vi "RM.forceAddReservation.vi"(5 "Resource Type":T1, 7 "Direction":T2, 8 "error in":errorcluster, 9 "reserver":string, 10 "name in bitfile":string, 11 "reservation DB in":variant) -> (0 "error out":errorcluster, 1 "replaced":bool, 3 "reservation DB out":variant)   [LabVIEW 2016, in "FPGA Addon Shared.lvlib"]
uses:
  FPGA Addon Shared.lvlib
  RM.resourceDirection.ctl
  RM.resourceType.ctl
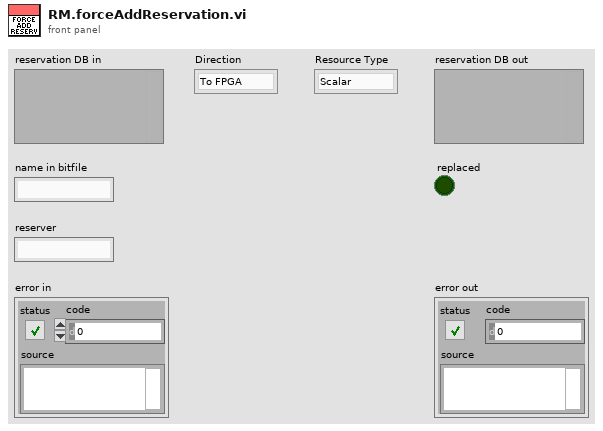
[diagram p1: front panel]
types:
  T1 = typedef "FPGA Addon Shared.lvlib/RM.resourceType.ctl" = enum16{"Scalar", "Waveform"}
  T2 = typedef "FPGA Addon Shared.lvlib/RM.resourceDirection.ctl" = enum16{"To FPGA", "From FPGA"}
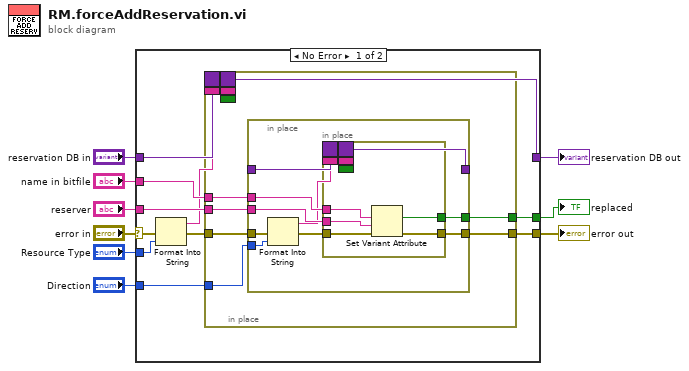
[diagram p0: block diagram]
diagram:
  n1 = case shown="No Error" "error in" {
    selector: "error in" -> [w12 w46]
    tunnel: "reservation DB in" -> [w20 w47]
    tunnel: "Direction" -> [w19 _]
    tunnel: [w18 w47] -> w7
    tunnel: "name in bitfile" -> [w17 _]
    tunnel: "reserver" -> [w16 _]
    tunnel: "Resource Type" -> [w15 _]
    tunnel: [w11 w46] -> w2
    tunnel: [w10 _] -> w1
    frame No Error {
      n2 = Format Into String(error in=w12, w15) -> (resulting string=w14:string, error out=w13:errorcluster)  [unwired: 2 in]
      n3 = in-place {
        border: w20 -> [_]
        border: w14 -> [_]
        border: [_] -> w18
        border: _ -> [_]
        border: _ -> [_]
        in-place-border: w19 -> [w28]
        in-place-border: w17 -> [w25]
        in-place-border: w16 -> [w24]
        in-place-border: w13 -> [w23]
        in-place-border: [w22] -> w11
        in-place-border: [w21] -> w10
        n4 = in-place {
          in-place-border: w28 -> [w34]
          in-place-border: w27 -> [w38]
          in-place-border: [w37] -> w26
          in-place-border: w25 -> [w36]
          in-place-border: w24 -> [w35]
          in-place-border: w23 -> [w32]
          in-place-border: [w30] -> w22
          in-place-border: [w29] -> w21
          n5 = Format Into String(error in=w32, w34) -> (resulting string=w33:string, error out=w31:errorcluster)  [unwired: 2 in]
          n6 = in-place {
            border: w38 -> [_]
            border: w33 -> [_]
            border: [_] -> w37
            border: _ -> [_]
            border: _ -> [_]
            in-place-border: w36 -> [w43]
            in-place-border: w35 -> [w42]
            in-place-border: w31 -> [w41]
            in-place-border: [w40] -> w30
            in-place-border: [w39] -> w29
            n7 = Set Variant Attribute(Variant=w45, name=w43, value=w42, error in=w41) -> (Variant out=w44:variant, replaced=w39:bool, error out=w40:errorcluster)
          }
        }
      }
    }
    frame Error {
    }
  }
  "reservation DB out" <- w7
  "error out" <- w2
  "replaced" <- w1
